vi "extractCollectionInformation.vi"(8 "error in (no error)":errorcluster, 10 "elementName":string, 11 "Topic in":refnum<class "Topic.lvclass">) -> (0 "error out":errorcluster, 2 "CollectionInfo":T1, 3 "Topic out":refnum<class "Topic.lvclass">)   [LabVIEW 2016, in "Topic.lvclass"]
uses:
  Topic.lvclass
  Typedefs/CollectionInfo.ctl
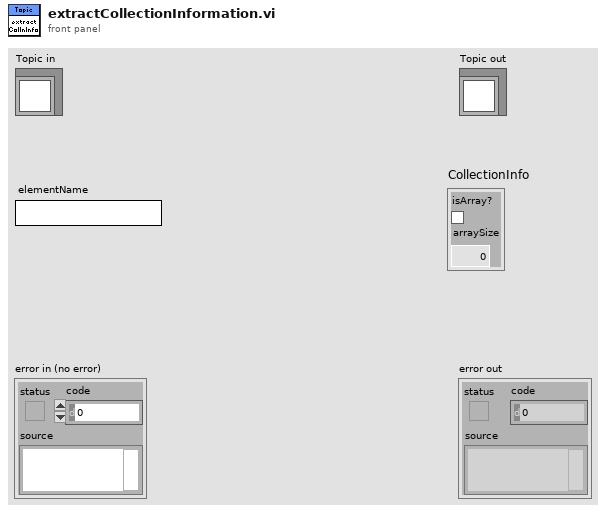
[diagram p1: front panel]
types:
  T1 = typedef "CollectionInfo.ctl" = cluster{"isArray?":bool, "arraySize":u16}
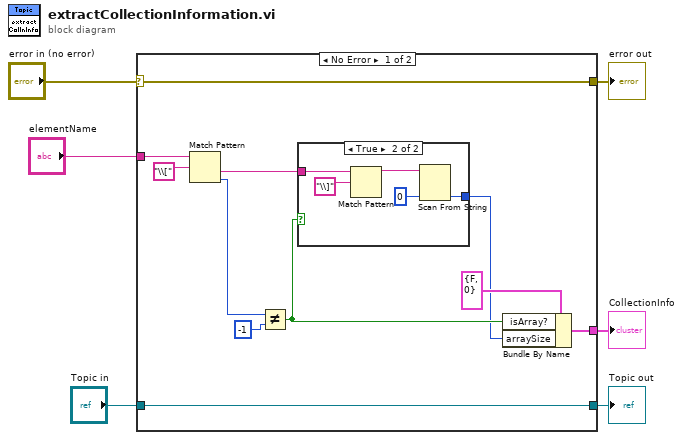
[diagram p0: block diagram]
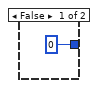
[diagram p2: hidden frame]
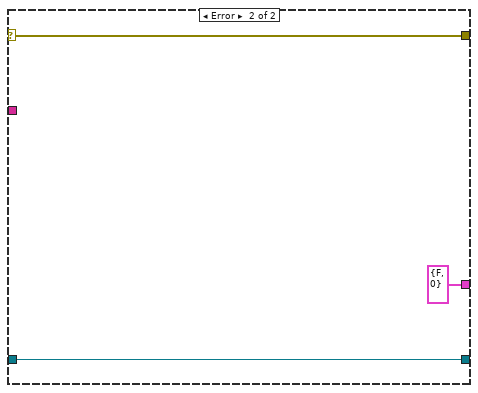
[diagram p3: hidden frame]
diagram:
  n1 = case shown="No Error" "error in (no error)" {
    selector: "error in (no error)" -> [w16 w26]
    tunnel: [w16 w26] -> w5
    tunnel: [w17 w25] -> w3
    tunnel: "Topic in" -> [w17 w25]
    tunnel: "elementName" -> [w12 _]
    tunnel: [w10 T1 {"isArray?"=FALSE, "arraySize"=0} ("CollectionInfo")] -> w1
    frame No Error {
      n2 = Match Pattern(string=w12, regular expression="\\[") -> (after substring=w8:string, offset past match=w14:i32)  [unwired: 1 in, 2 out]
      n3 = Not Equal?(x=w14, y=-1) -> (x != y?=w9:bool)
      n4 = case shown="True" w9 {
        tunnel: w8 -> [_ w22]
        tunnel: [u16 0 ("arraySize") w19] -> w7
        frame False {
        }
        frame True {
          n5 = Match Pattern(string=w22, regular expression="\\]") -> (before substring=w21:string)  [unwired: 1 in, 3 out]
          n6 = Scan From String(input string=w21, default 1=u16 0 ("arraySize")) -> (output 1=w19:u16)  [unwired: 3 in, 3 out]
        }
      }
      n7 = Bundle By Name(cluster=T1 {"isArray?"=FALSE, "arraySize"=0} ("CollectionInfo"), "isArray?"=w9, "arraySize"=w7) -> (w10:T1)
    }
    frame Error {
    }
  }
  "error out" <- w5
  "Topic out" <- w3
  "CollectionInfo" <- w1
